vi "SerialSubroutine.vi"() -> ()   [LabVIEW 2010]
panel:
  out "error":errorcluster
  in  "error IO":errorcluster
  in  "Command":string
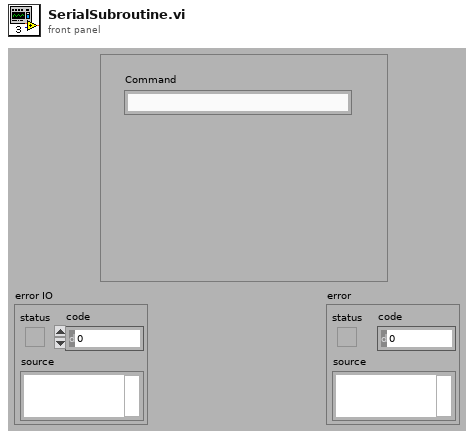
[diagram p1: front panel]
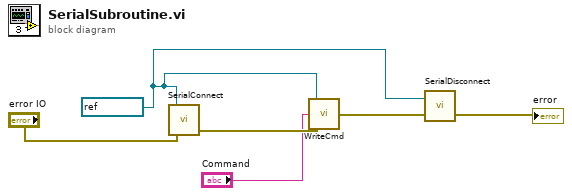
[diagram p0: block diagram]
diagram:
  w1 = refnum<visa-resource-name> "COM3" ("VISA resource name")
  n1 = call "SerialConnect.vi"("error in (no error)"="error IO", "VISA resource name"=w1) -> ("error out"=w6:errorcluster)  [unwired: 3 in]
  n2 = call "WriteCmd.vi"("error IO"=w6, "Command"="Command", "VISA resource name"=w1) -> ("error"=w4:errorcluster)
  n3 = call "SerialDisconnect.vi"("error in (no error)"=w4, "VISA resource name"=w1) -> ("error out"=→"error":errorcluster)  [unwired: 1 in]
